vi "Parse API Responce Body.vi"(8 "error in (no error)":errorcluster, 10 "Body Parameters Names in":string[](array[string]), 11 "Response Body in":string) -> (0 "error out":errorcluster, 2 "Body Parameters out":T1[](array[typedef]), 3 "Response Body out":string)   [LabVIEW 2019]
uses:
  Types/Body Parameter Type.ctl
  <vilib>/LVH/i3 JSON/JSON Parsing/Get Object Parameter Files/Get Object Parameter - String.vi
  <vilib>/LVH/i3 JSON/i3-json.lvlib
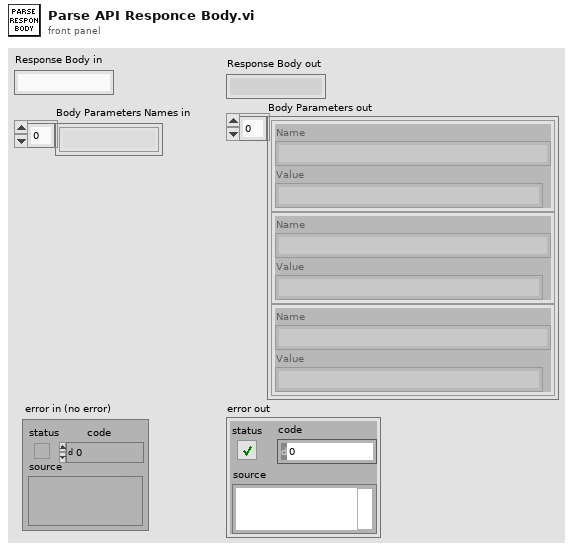
[diagram p1: front panel]
types:
  T1 = typedef "Body Parameter Type.ctl" = cluster{"Name":string, "Value":string}
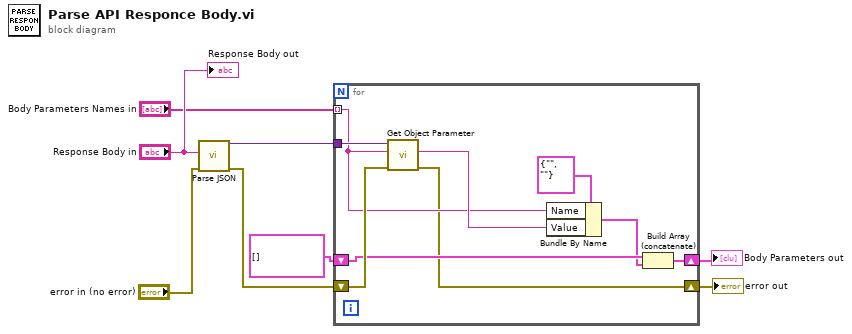
[diagram p0: block diagram]
diagram:
  n1 = call <vilib>:"Parse JSON.vi"("error in (no error)"="error in (no error)", "JSON String"="Response Body in") -> ("error out"=w6:errorcluster, "JSON Tree"=w8:variant)  [unwired: 6 in, 2 out]
  n2 = for {
    tunnel: w8 -> [w17]
    tunnel: "Body Parameters Names in" -> [w13] mode=indexing
    shift-right: [w9] -> w2
    shift-left: w6 -> [w16]
    shift-right: [w10] -> w1
    shift-left: T1[] [] -> [w12]
    n3 = call-poly <vilib>:"Get Object Parameter.vi"("error in (no error)"=w16, "Parameter Name"=w13, "JSON Tree In (JSON Object)"=w17) -> ("error out"=w9:errorcluster, "String Value"=w15:string)  [unwired: 5 in, 2 out]
    n4 = Bundle By Name(cluster=T1 {"Name"="", "Value"=""} ("Body Parameter"), "Name"=w13, "Value"=w15) -> (w11:T1)
    n5 = Build Array (concatenate)(w12, w11) -> (w10:T1[])
  }
  "error out" <- w2
  "Body Parameters out" <- w1
  "Response Body out" <- "Response Body in"
